vi "Check and set PID.vi"(8 "Error In":errorcluster, 9 "Old data":T1={"Channels to measure"=[1.0], "Record heater"=FALSE, "Set point"=0.0, "Set Heater Range"=enum."Off", "Control"=FALSE, "Approach"=enum."Instant", "Ramp rate, K/min"=1.0, "Control Channel"=1, "P"=0.0, "I"=0.0, "D"=0.0, "Suspend heater"=FALSE}, 10 "New data":T1={"Channels to measure"=[1.0], "Record heater"=FALSE, "Set point"=0.0, "Set Heater Range"=enum."Off", "Control"=FALSE, "Approach"=enum."Instant", "Ramp rate, K/min"=1.0, "Control Channel"=1, "P"=0.0, "I"=0.0, "D"=0.0, "Suspend heater"=FALSE}, 11 "VISA resource name":refnum<visa-resource-name>) -> (0 "Error Out":errorcluster, 3 "VISA resource name out":refnum<visa-resource-name>)   [LabVIEW 2015]
uses:
  Neocera Front Panel Data.ctl
  Neocera Heater Ranges.ctl
  Neocera Set Point Aproach.ctl
panel:
  # "Temperature Monitor"
  # "Temperature Control"
  # "Temperature Monitor"
  # "Temperature Control"
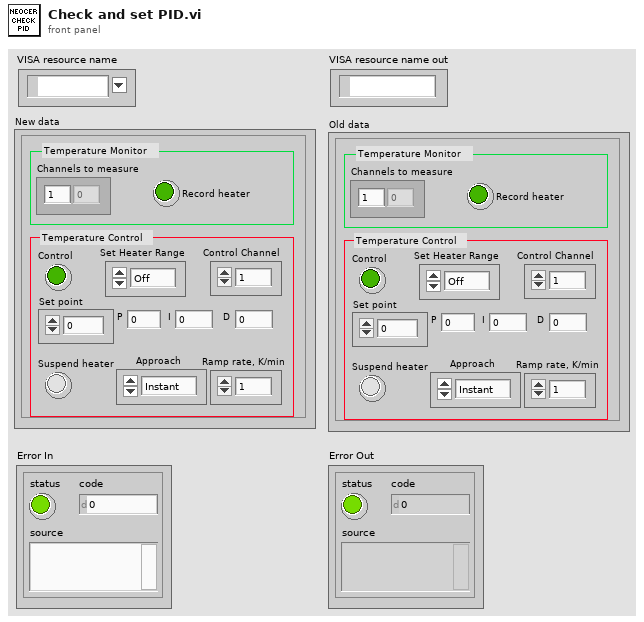
[diagram p1: front panel]
types:
  T1 = typedef "Neocera Front Panel Data.ctl" = cluster{"Channels to measure":dbl[], "Record heater":bool, "Set point":dbl, "Set Heater Range":T2, "Control":bool, "Approach":T3, "Ramp rate, K/min":dbl, "Control Channel":i16, "P":dbl, "I":dbl, "D":dbl, "Suspend heater":bool}
  T2 = typedef "Neocera Heater Ranges.ctl" = enum16{"Off", "0.05W", "0.5W", "5W", "50W"}
  T3 = typedef "Neocera Set Point Aproach.ctl" = enum16{"Instant", "Ramp"}
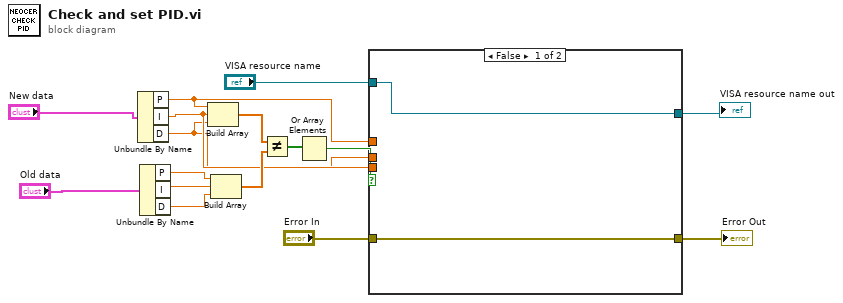
[diagram p0: block diagram]
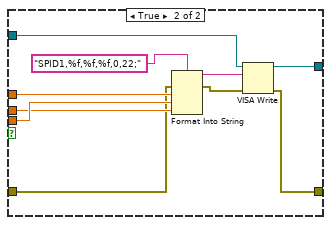
[diagram p2: hidden frame]
diagram:
  n1 = Unbundle By Name("New data") -> ("P"=w7:dbl, "I"=w6:dbl, "D"=w5:dbl)
  n2 = Unbundle By Name("Old data") -> ("P"=w14:dbl, "I"=w13:dbl, "D"=w12:dbl)
  n3 = Build Array(w7, w6, w5) -> (w11:dbl[])
  n4 = Build Array(w14, w13, w12) -> (w10:dbl[])
  n5 = Not Equal?(x=w11, y=w10) -> (x != y?=w9:bool[])
  n6 = Or Array Elements(Boolean array=w9) -> (logical OR=w8:bool)
  n7 = case shown="False" w8 {
    tunnel: w7 -> [_ w27]
    tunnel: w6 -> [_ w26]
    tunnel: w5 -> [_ w25]
    tunnel: "Error In" -> [w17 w24]
    tunnel: [w17 w19] -> w3
    tunnel: "VISA resource name" -> [w18 w21]
    tunnel: [w18 w20] -> w1
    frame False {
    }
    frame True {
      n8 = Format Into String(format string="SPID1,%f,%f,%f,0,22;", error in=w24, w27, w26, w25) -> (resulting string=w22:string, error out=w23:errorcluster)  [unwired: 1 in]
      n9 = VISA Write(VISA resource name=w21, write buffer=w22, error in (no error)=w23) -> (VISA resource name out=w20:refnum<visa-resource-name>, error out=w19:errorcluster)  [unwired: 1 out]
    }
  }
  "VISA resource name out" <- w1
  "Error Out" <- w3
